vi "main_picometerControl1.vi"() -> ()   [LabVIEW 2018]
uses:
  Device VIs/Verbal.vi
panel:
  out "空闲":bool
  in  "单步时间ms":u32=100
  in  "CH2归0":bool
  in  "CH1归0":bool
  out "OK":bool
  in  "制动":bool
  in  "CH2启动":bool
  in  "CH1启动":bool
  in  "CH2 运动步数":i32
  in  "CH1 运动步数":i32
  out "CH2 当前位置":i32
  out "CH1 当前位置":i32
  out "状态":string
  out "error out":errorcluster
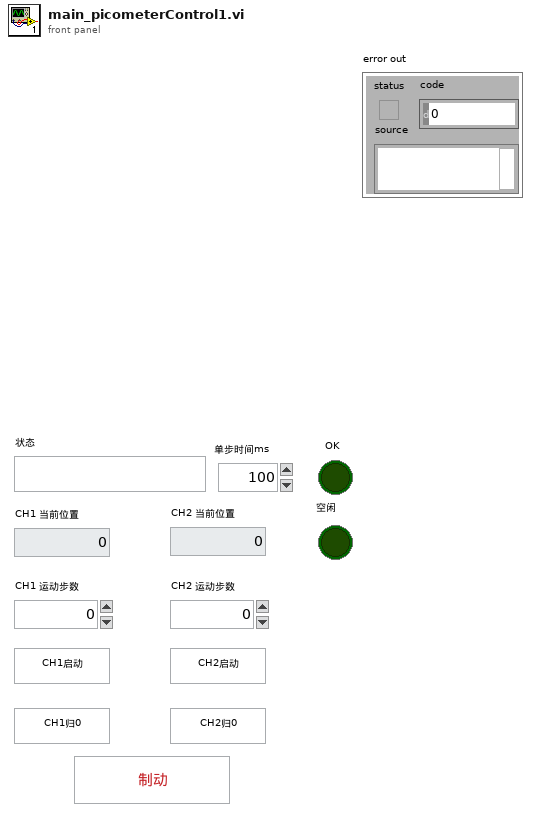
[diagram p1: front panel]
types:
  T1 = cluster{"DeviceKey":string, "Device Address":i32, "Controller Name":string}[]
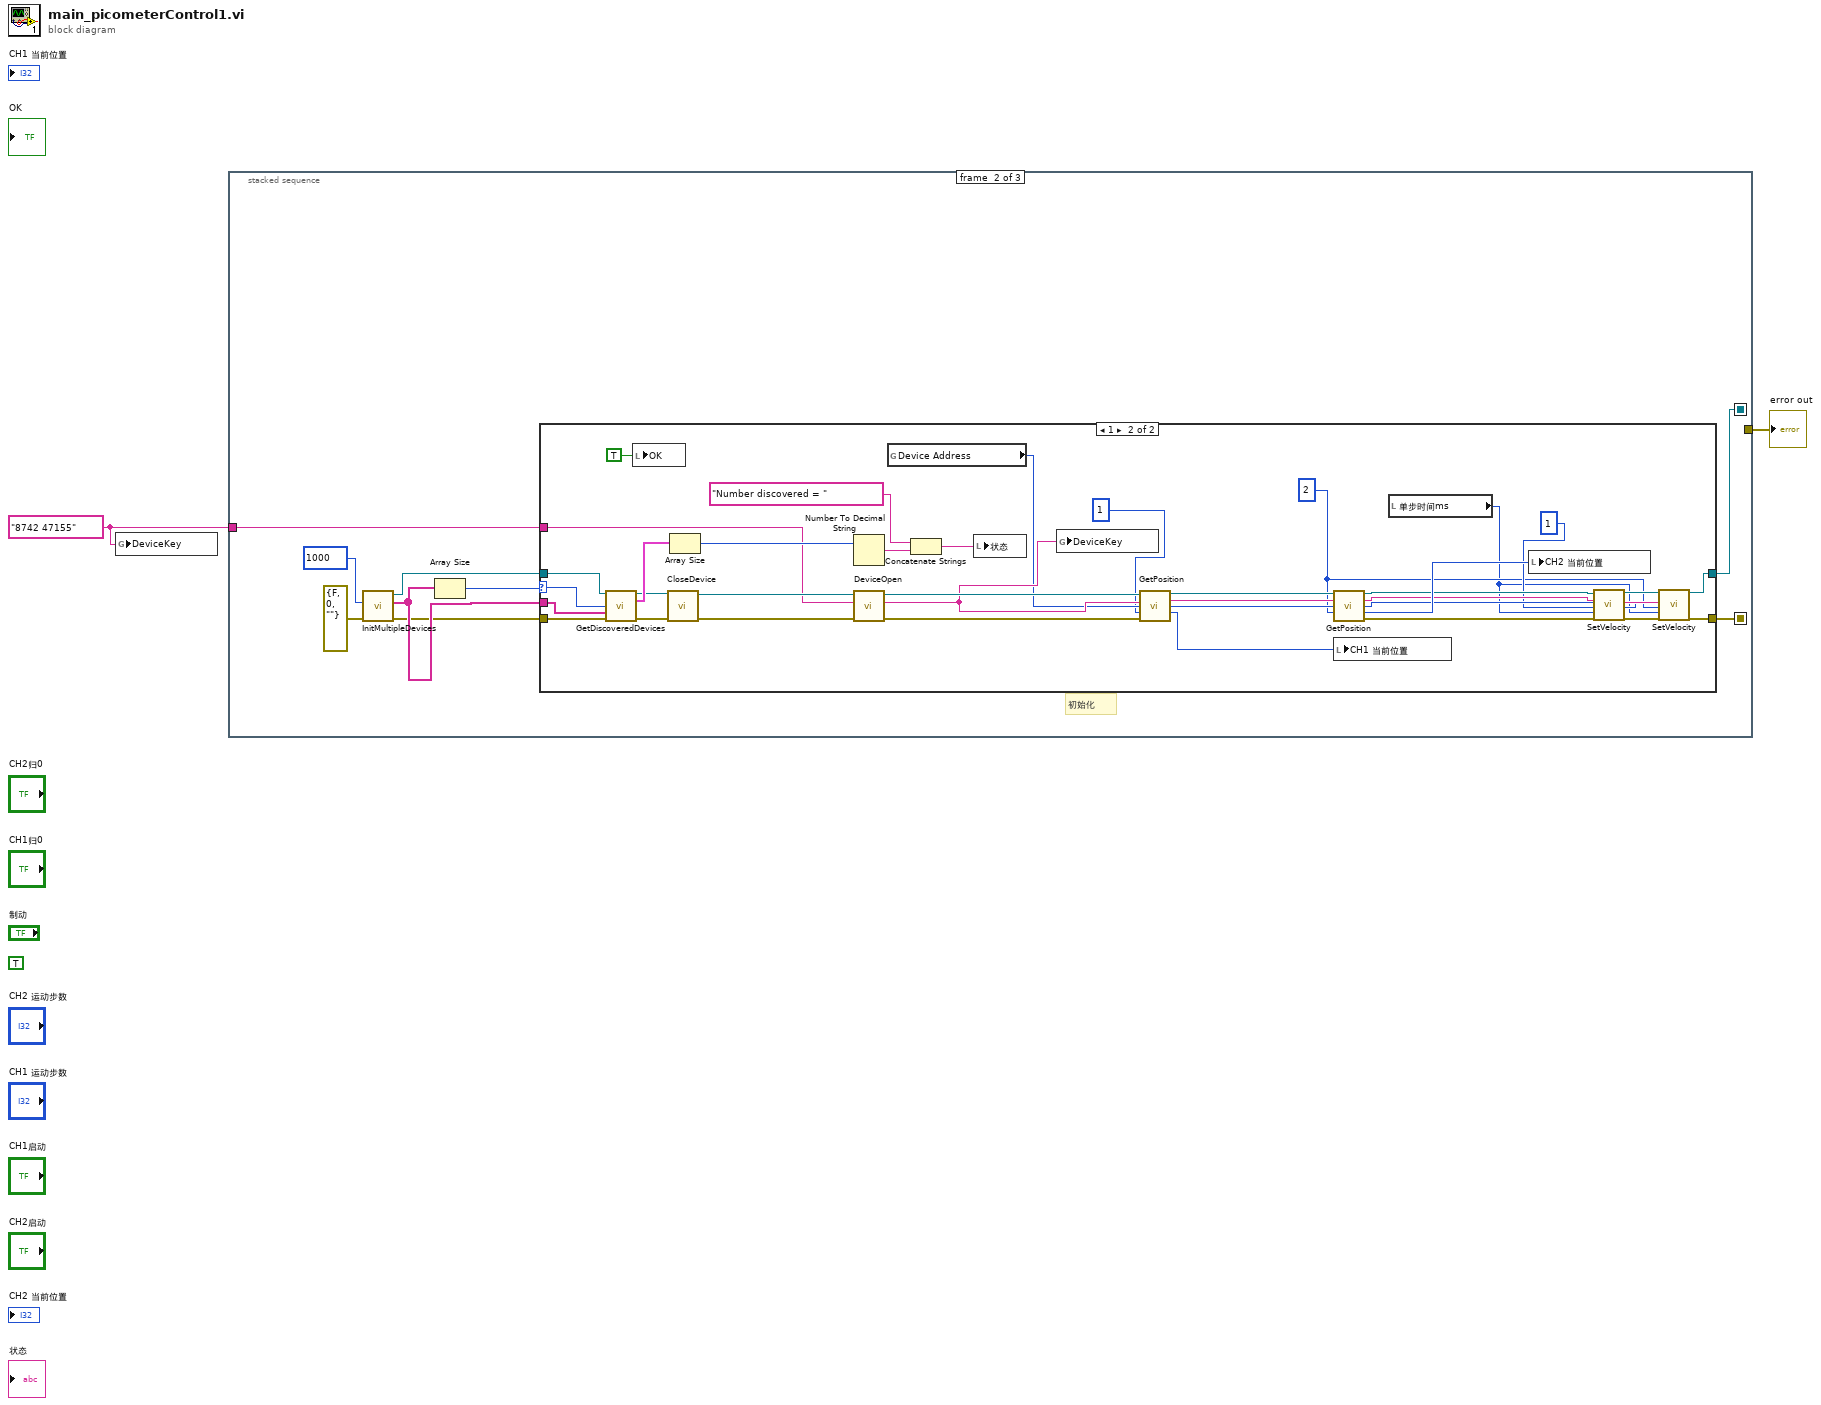
[diagram p0: block diagram]
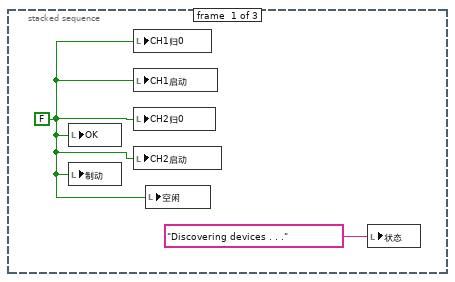
[diagram p2: hidden frame]
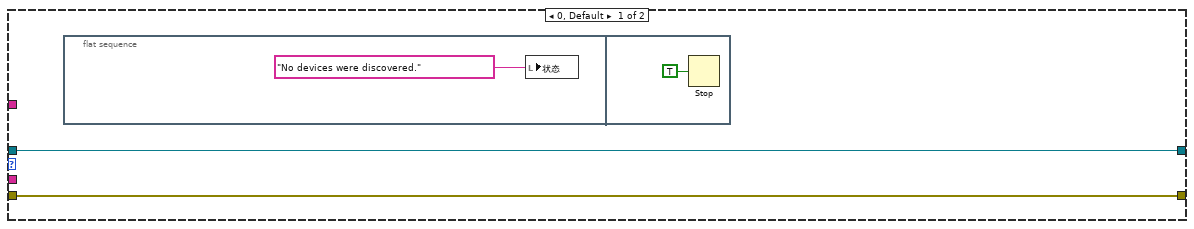
[diagram p3: hidden frame]
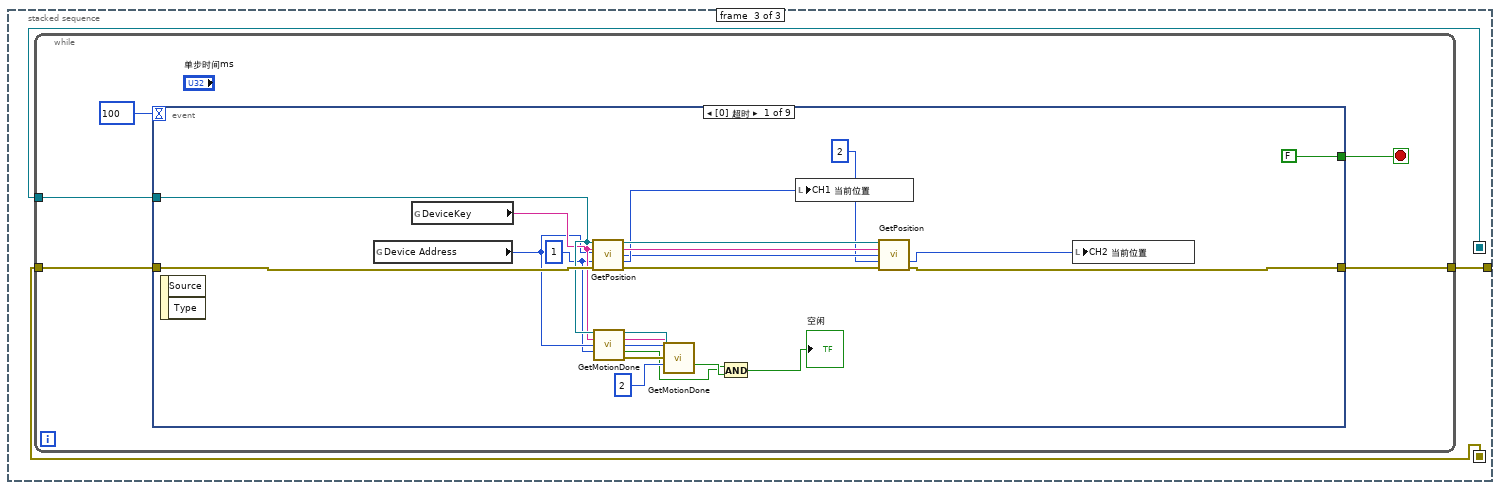
[diagram p4: hidden frame]
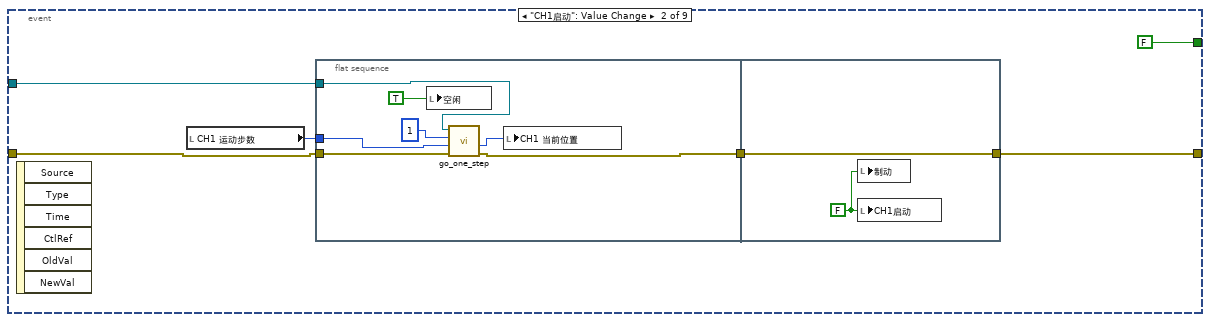
[diagram p5: hidden frame]
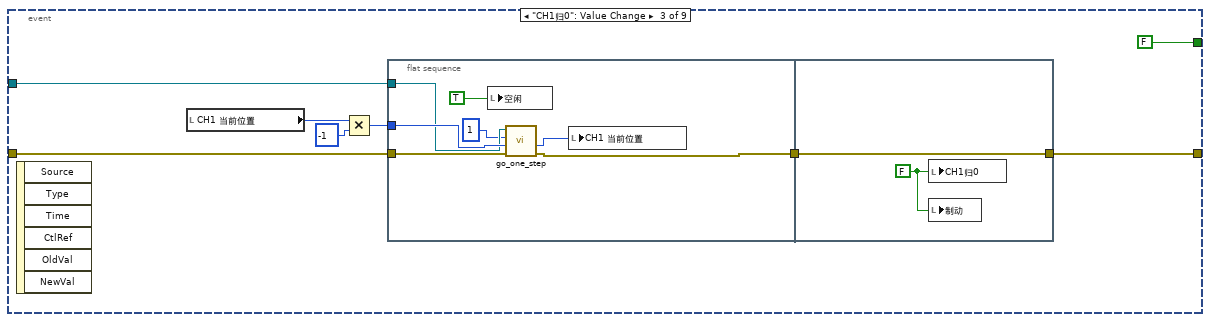
[diagram p6: hidden frame]
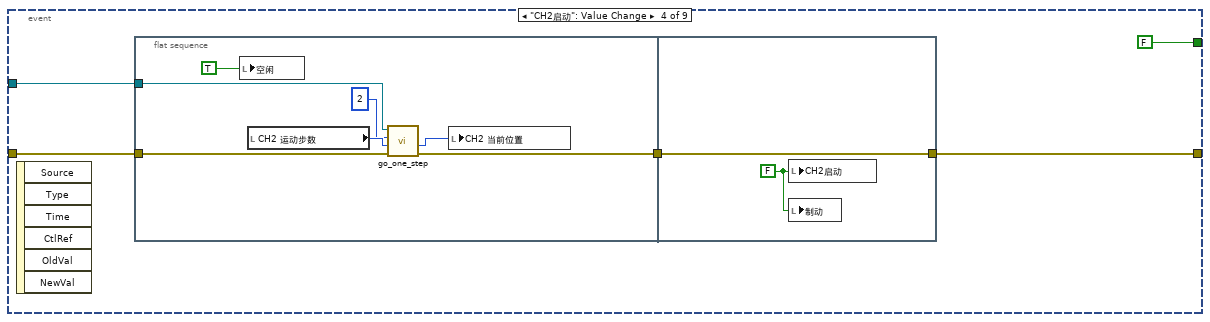
[diagram p7: hidden frame]
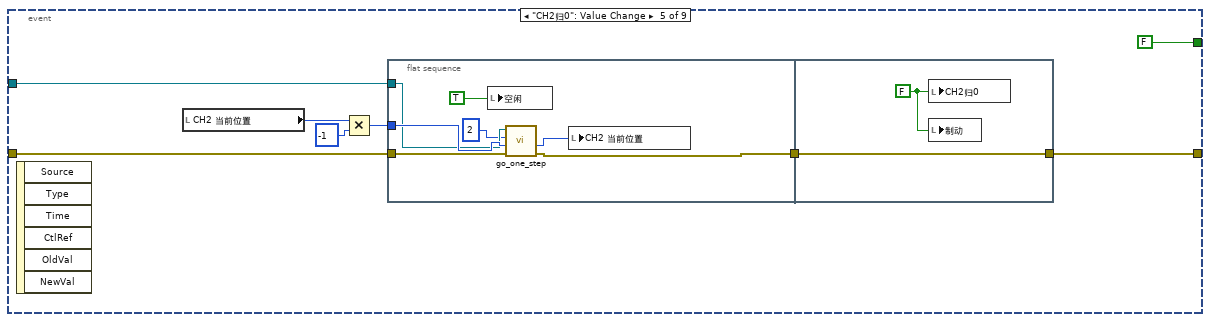
[diagram p8: hidden frame]
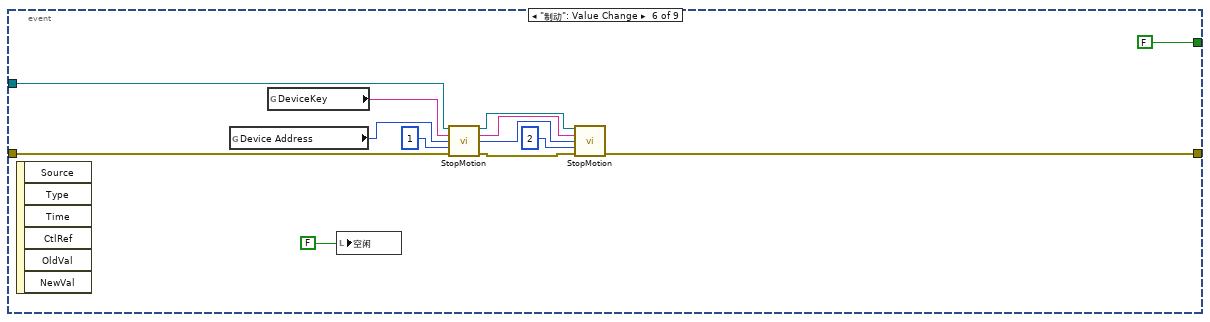
[diagram p9: hidden frame]
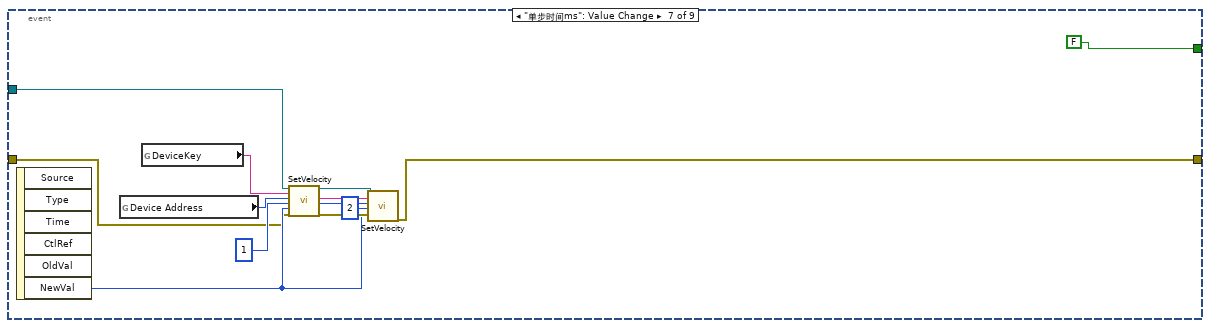
[diagram p10: hidden frame]
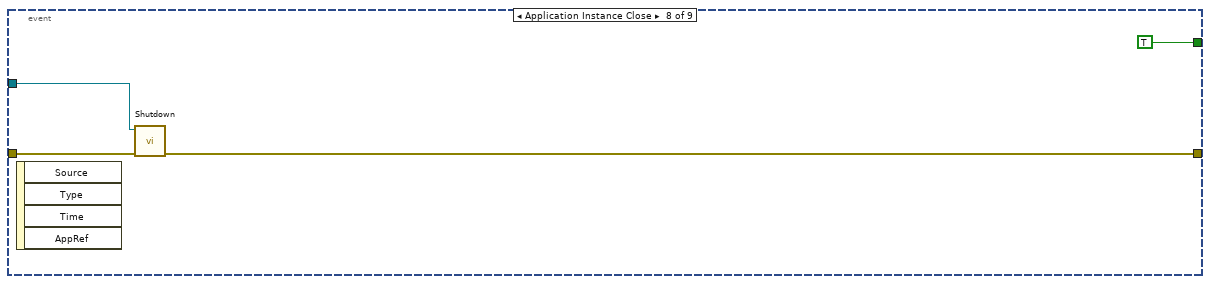
[diagram p11: hidden frame]
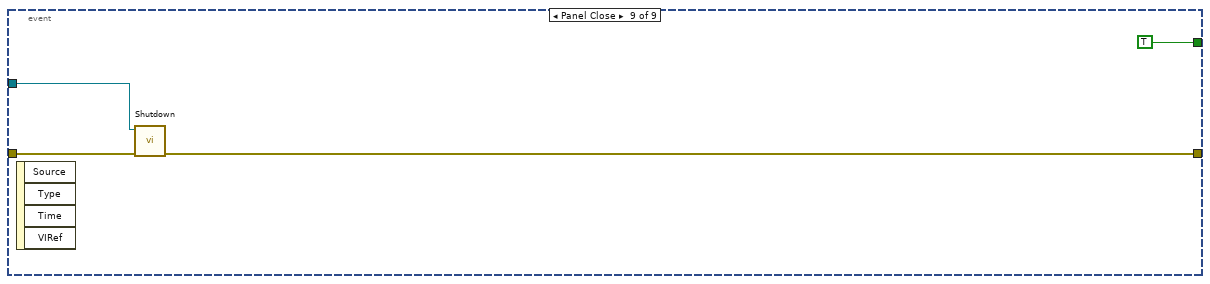
[diagram p12: hidden frame]
diagram:
  (unwired) TRUE
  w2 = "8742 47155" ("Message")
  n1 = global write "Verbal.vi" "DeviceKey"(w2) -> ()
  n2 = stacked-sequence {
    seq-local: [_ w6 _] -> [_ _ w58]
    seq-local: [_ w5 _] -> [_ _ w57]
    tunnel: w2 -> [_ w7 _]
    tunnel: [_ _ w56] -> w1
    frame #0 {
      w3 = FALSE ("Motion")
      n3 = local write "OK"(w3) -> ()
      n4 = local write "制动"(w3) -> ()
      n5 = local write "CH1归0"(w3) -> ()
      n6 = local write "CH1启动"(w3) -> ()
      n7 = local write "CH2归0"(w3) -> ()
      n8 = local write "CH2启动"(w3) -> ()
      n9 = local write "空闲"(w3) -> ()
      n10 = local write "状态"("Discovering devices . . ." ("Message")) -> ()
    }
    frame #1 {
      # "初始化"
      n11 = call "InitMultipleDevices.vi"("error in (no error)"=errorcluster {"status"=FALSE, "code"=0, "source"=""}, "msecDelayForDiscovery"=1000) -> ("error out"=w8:errorcluster, "DeviceKey List Out"=w9:string[], "CmdLib Out"=w10:refnum<k24>)  [unwired: 3 in]
      n12 = Array Size(array=w9) -> (size(s)=w11:i32)
      n13 = case shown="1" w11 {
        selector: w11 -> [_ w51]
        tunnel: w10 -> [w15 w52]
        tunnel: w9 -> [_ w50]
        tunnel: w8 -> [w14 w49]
        tunnel: w7 -> [_ w45]
        tunnel: [w15 w18] -> w6
        tunnel: [w14 w19] -> w5
        frame 0, Default {
          n14 = flat-sequence {
            frame #0 {
              n15 = local write "状态"("No devices were discovered." ("Input String")) -> ()
            }
            frame #1 {
              n16 = Stop(stop? (T)=TRUE ("停止？(T)")) -> ()
            }
          }
        }
        frame 1 {
          w22 = 2 ("Motor")
          n17 = call "GetDiscoveredDevices.vi"("CmdLib In"=w52, "Master Count"=w51, "DeviceKey List"=w50, "error in"=w49) -> ("CmdLib Out"=w47:refnum<k24>, "Device Array"=w48:T1, "error out"=w44:errorcluster)  [unwired: 9 in]
          n18 = local write "OK"(TRUE ("等待指令")) -> ()
          n19 = call "CloseDevice.vi"("error in"=w44, "CmdLib In"=w47) -> ("error out"=w43:errorcluster, "CmdLib Out"=w46:refnum<k24>)  [unwired: 8 in]
          n20 = Array Size(array=w48) -> (size(s)=w55:i32)
          n21 = Number To Decimal String(number=w55) -> (decimal integer string=w53:string)  [unwired: 1 in]
          n22 = call "DeviceOpen.vi"("error in (no error)"=w43, "DeviceKey In"=w45, "CmdLib In"=w46) -> ("error out"=w38:errorcluster, "DeviceKey Out"=w41:string, "CmdLib Out"=w42:refnum<k24>)  [unwired: 2 in]
          n23 = global read "Verbal.vi" "Device Address"() -> (w40:i32)
          n24 = Concatenate Strings("Number discovered = " ("string"), w53) -> (w32:string)
          n25 = local write "状态"(w32) -> ()
          n26 = global write "Verbal.vi" "DeviceKey"(w41) -> ()
          n27 = call "GetPosition.vi"("CmdLib In"=w42, "DeviceKey In"=w41, "Device Address In"=w40, "Motor"=1, "error in (no error)"=w38) -> ("CmdLib Out"=w36:refnum<k24>, "DeviceKey Out"=w35:string, "Device Address Out"=w34:i32, "Position"=w37:i32)  [unwired: 6 in, 1 out]
          n28 = call "GetPosition.vi"("CmdLib In"=w36, "DeviceKey In"=w35, "Device Address In"=w34, "Motor"=w22) -> ("CmdLib Out"=w30:refnum<k24>, "DeviceKey Out"=w29:string, "Device Address Out"=w28:i32, "Position"=w33:i32, "error out"=w26:errorcluster)  [unwired: 7 in]
          n29 = local write "CH1 当前位置"(w37) -> ()
          n30 = local read "单步时间ms"() -> (w21:u32)
          n31 = local write "CH2 当前位置"(w33) -> ()
          n32 = call "SetVelocity.vi"("CmdLib In"=w30, "DeviceKey In"=w29, "Device Address In"=w28, "Motor"=1, "Steps Per Sec"=w21, "error in (no error)"=w26) -> ("CmdLib Out"=w25:refnum<k24>, "DeviceKey Out"=w24:string, "Device Address Out"=w23:i32, "error out"=w20:errorcluster)  [unwired: 10 in]
          n33 = call "SetVelocity.vi"("CmdLib In"=w25, "DeviceKey In"=w24, "Device Address In"=w23, "Motor"=w22, "Steps Per Sec"=w21, "error in (no error)"=w20) -> ("CmdLib Out"=w18:refnum<k24>, "error out"=w19:errorcluster)  [unwired: 10 in, 2 out]
        }
      }
    }
    frame #2 {
      n34 = while {
        tunnel: w58 -> [w62]
        tunnel: w57 -> [w61]
        tunnel: [w60] -> w56
        stop <- w59 stop-if-true
        n35 = event shown="[0] 超时" {
          selector: _ -> [_ _ _ _ _ _ _ _ _]
          dyn-events: _ -> [_ _ _ _ _ _ _ _ _]
          timeout: 100 -> [_ _ _ _ _ _ _ _ _]
          tunnel: w62 -> [w75 w91 w105 w122 w136 w159 w169 w178 w182]
          tunnel: w61 -> [w78 w90 w104 w120 w135 w160 w164 w177 w181]
          tunnel: [w76 w89 w102 w121 w134 w150 w163 w176 w180] -> w60
          tunnel: [FALSE FALSE FALSE FALSE FALSE FALSE FALSE TRUE TRUE] -> w59
          event Timeout {
            w72 = 1 ("Motor")
            n36 = event-data() -> ()  [unwired: 1 in, 2 out]
            n37 = global read "Verbal.vi" "Device Address"() -> (w73:i32)
            n38 = global read "Verbal.vi" "DeviceKey"() -> (w74:string)
            n39 = call "GetPosition.vi"("CmdLib In"=w75, "DeviceKey In"=w74, "Device Address In"=w73, "Motor"=w72, "error in (no error)"=w78) -> ("CmdLib Out"=w85:refnum<k24>, "DeviceKey Out"=w84:string, "Device Address Out"=w82:i32, "Position"=w83:i32, "error out"=w77:errorcluster)  [unwired: 6 in]
            n40 = call "GetMotionDone.vi"("CmdLib In"=w75, "DeviceKey In"=w74, "Device Address In"=w73, "Motor"=w72) -> ("CmdLib Out"=w70:refnum<k24>, "DeviceKey Out"=w69:string, "Device Address Out"=w68:i32, "Is Motion Done"=w64:bool, "error out"=w67:errorcluster)  [unwired: 7 in]
            n41 = call "GetMotionDone.vi"("CmdLib In"=w70, "DeviceKey In"=w69, "Device Address In"=w68, "Motor"=2, "error in (no error)"=w67) -> ("Is Motion Done"=w65:bool)  [unwired: 6 in, 4 out]
            n42 = And(x=w64, y=w65) -> (x .and. y?=→"空闲":bool)
            n43 = local write "CH1 当前位置"(w83) -> ()
            n44 = call "GetPosition.vi"("CmdLib In"=w85, "DeviceKey In"=w84, "Device Address In"=w82, "Motor"=2, "error in (no error)"=w77) -> ("Position"=w80:i32, "error out"=w76:errorcluster)  [unwired: 6 in, 3 out]
            n45 = local write "CH2 当前位置"(w80) -> ()
          }
          event "CH1启动": Value Change {
            n46 = event-data() -> ()  [unwired: 1 in, 6 out]
            n47 = local read "CH1 运动步数"() -> (w87:i32)
            n48 = flat-sequence {
              tunnel: w91 -> [w98]
              tunnel: w90 -> [w97]
              tunnel: w87 -> [w95]
              tunnel: [w96] -> w86
              tunnel: [w100] -> w89
              tunnel: w86 -> [w100]
              frame #0 {
                n49 = local write "空闲"(TRUE ("Motion")) -> ()
                n50 = call "go_one_step.vi"("error in"=w97, "Step"=w95, "Motor"=1, "CmdLib In"=w98) -> ("error out"=w96:errorcluster, "Position"=w92:i32)  [unwired: 1 in, 1 out]
                n51 = local write "CH1 当前位置"(w92) -> ()
              }
              frame #1 {
                w99 = FALSE ("制动")
                n52 = local write "制动"(w99) -> ()
                n53 = local write "CH1启动"(w99) -> ()
              }
            }
          }
          event "CH1归0": Value Change {
            n54 = event-data() -> ()  [unwired: 1 in, 6 out]
            n55 = local read "CH1 当前位置"() -> (w108:i32)
            n56 = Multiply(x=w108, y=-1) -> (x*y=w106:i32)
            n57 = flat-sequence {
              tunnel: w106 -> [w115]
              tunnel: w105 -> [w114]
              tunnel: w104 -> [w113]
              tunnel: [w112] -> w101
              tunnel: [w117] -> w102
              tunnel: w101 -> [w117]
              frame #0 {
                n58 = local write "空闲"(TRUE ("Motion")) -> ()
                n59 = call "go_one_step.vi"("error in"=w113, "Step"=w115, "Motor"=1, "CmdLib In"=w114) -> ("error out"=w112:errorcluster, "Position"=w109:i32)  [unwired: 1 in, 1 out]
                n60 = local write "CH1 当前位置"(w109) -> ()
              }
              frame #1 {
                w116 = FALSE ("制动")
                n61 = local write "CH1归0"(w116) -> ()
                n62 = local write "制动"(w116) -> ()
              }
            }
          }
          event "CH2启动": Value Change {
            n63 = event-data() -> ()  [unwired: 1 in, 6 out]
            n64 = flat-sequence {
              tunnel: w122 -> [w129]
              tunnel: w120 -> [w126]
              tunnel: [w127] -> w118
              tunnel: [w131] -> w121
              tunnel: w118 -> [w131]
              frame #0 {
                n65 = local write "空闲"(TRUE ("Motion")) -> ()
                n66 = local read "CH2 运动步数"() -> (w128:i32)
                n67 = call "go_one_step.vi"("error in"=w126, "Step"=w128, "Motor"=2, "CmdLib In"=w129) -> ("error out"=w127:errorcluster, "Position"=w123:i32)  [unwired: 1 in, 1 out]
                n68 = local write "CH2 当前位置"(w123) -> ()
              }
              frame #1 {
                w130 = FALSE
                n69 = local write "CH2启动"(w130) -> ()
                n70 = local write "制动"(w130) -> ()
              }
            }
          }
          event "CH2归0": Value Change {
            n71 = event-data() -> ()  [unwired: 1 in, 6 out]
            n72 = local read "CH2 当前位置"() -> (w139:i32)
            n73 = Multiply(x=w139, y=-1) -> (x*y=w137:i32)
            n74 = flat-sequence {
              tunnel: w137 -> [w146]
              tunnel: w136 -> [w145]
              tunnel: w135 -> [w144]
              tunnel: [w143] -> w132
              tunnel: [w148] -> w134
              tunnel: w132 -> [w148]
              frame #0 {
                n75 = local write "空闲"(TRUE ("Motion")) -> ()
                n76 = call "go_one_step.vi"("error in"=w144, "Step"=w146, "Motor"=2, "CmdLib In"=w145) -> ("error out"=w143:errorcluster, "Position"=w140:i32)  [unwired: 1 in, 1 out]
                n77 = local write "CH2 当前位置"(w140) -> ()
              }
              frame #1 {
                w147 = FALSE ("制动")
                n78 = local write "CH2归0"(w147) -> ()
                n79 = local write "制动"(w147) -> ()
              }
            }
          }
          event "制动": Value Change {
            n80 = event-data() -> ()  [unwired: 1 in, 6 out]
            n81 = global read "Verbal.vi" "Device Address"() -> (w157:i32)
            n82 = global read "Verbal.vi" "DeviceKey"() -> (w158:string)
            n83 = local write "空闲"(FALSE ("Motion")) -> ()
            n84 = call "StopMotion.vi"("CmdLib In"=w159, "DeviceKey In"=w158, "Device Address In"=w157, "Motor"=1, "error in (no error)"=w160) -> ("CmdLib Out"=w155:refnum<k24>, "DeviceKey Out"=w154:string, "Device Address Out"=w153:i32, "error out"=w151:errorcluster)  [unwired: 7 in]
            n85 = call "StopMotion.vi"("CmdLib In"=w155, "DeviceKey In"=w154, "Device Address In"=w153, "Motor"=2, "error in (no error)"=w151) -> ("error out"=w150:errorcluster)  [unwired: 7 in, 3 out]
          }
          event "单步时间ms": Value Change {
            n86 = event-data() -> ("NewVal"=w165:u32)  [unwired: 1 in, 5 out]
            n87 = global read "Verbal.vi" "Device Address"() -> (w168:i32)
            n88 = global read "Verbal.vi" "DeviceKey"() -> (w170:string)
            n89 = call "SetVelocity.vi"("CmdLib In"=w169, "DeviceKey In"=w170, "Device Address In"=w168, "Motor"=1, "Steps Per Sec"=w165, "error in (no error)"=w164) -> ("CmdLib Out"=w174:refnum<k24>, "DeviceKey Out"=w173:string, "Device Address Out"=w171:i32, "error out"=w172:errorcluster)  [unwired: 10 in]
            n90 = call "SetVelocity.vi"("CmdLib In"=w174, "DeviceKey In"=w173, "Device Address In"=w171, "Motor"=2, "Steps Per Sec"=w165, "error in (no error)"=w172) -> ("error out"=w163:errorcluster)  [unwired: 10 in, 3 out]
          }
          event Application Instance Close {
            n91 = event-data() -> ()  [unwired: 1 in, 4 out]
            n92 = call "Shutdown.vi"("error in (no error)"=w177, "CmdLib In"=w178) -> ("error out"=w176:errorcluster)  [unwired: 4 in, 1 out]
          }
          event Panel Close {
            n93 = event-data() -> ()  [unwired: 1 in, 4 out]
            n94 = call "Shutdown.vi"("error in (no error)"=w181, "CmdLib In"=w182) -> ("error out"=w180:errorcluster)  [unwired: 4 in, 1 out]
          }
        }
      }
    }
  }
  "error out" <- w1
